vi "Main_Robot_Control.vi"() -> ()   [LabVIEW 2014]
uses:
  <instrlib>/Hokuyo URG Series/Public/Initialize-Standard.vi
  <instrlib>/Hokuyo URG Series/Hokuyo URG Series.lvlib
panel:
  in  "stop 2":bool
  in  "polar attributes (hidden)":T1={"maximum"=30000.0, "minimum"=0.0, "clip to min"=FALSE, "log?(F)"=TRUE, "grid color"=6710886, "plot color"=65280, "fmt and prec"={"format"=enum."Decimal", "precision"=0}, "visible section"=8} {"minimum" format="%0.2f"; "maximum" format="%0.2f"}
  in  "Tab Control":T2(tab)
  out "?":dbl(knob) scale=-800.0..800.0
  out "Sensor Head Position":dbl
  out "Blinky Light":bool
  out "Stop Engaged":bool
  in  "?":bool
  out "Raw Volts":dbl
  out "Center_JR":dbl(slide) scale=0.0..3.0
  out "Pot":dbl(slide) min=0.0 max=5.0 step=0.25 scale=0.0..5.0
  in  "Motor Direction":bool
  in  "1) SET Start Position of Head":dbl
  in  "stop":bool
  out "IR_V":dynamicdata(graph)
  out "Pot_V":dynamicdata(graph)
  out "IR_D":dynamicdata(graph)
  out "Pot_D":dynamicdata(graph)
  out "Data Aquired":picture
  out "Blinky LIDAR  Running":bool
  in  "VISA resource name":refnum<visa-resource-name>="COM3"
  in  "Encoding Width":u16(ring)=3 items=["2 Byte"=2, "3 Byte"=3]
  in  "Cluster Count":dbl=1.0
  in  "Start Point":dbl=-50.0
  in  "End Point":dbl=33.0
  in  "Max (m)":dbl=1.0
  in  "Plot Color":u32(colorbox)=14422272
  in  "Grid Color":u32(colorbox)=11776947
  in  "Stop":bool
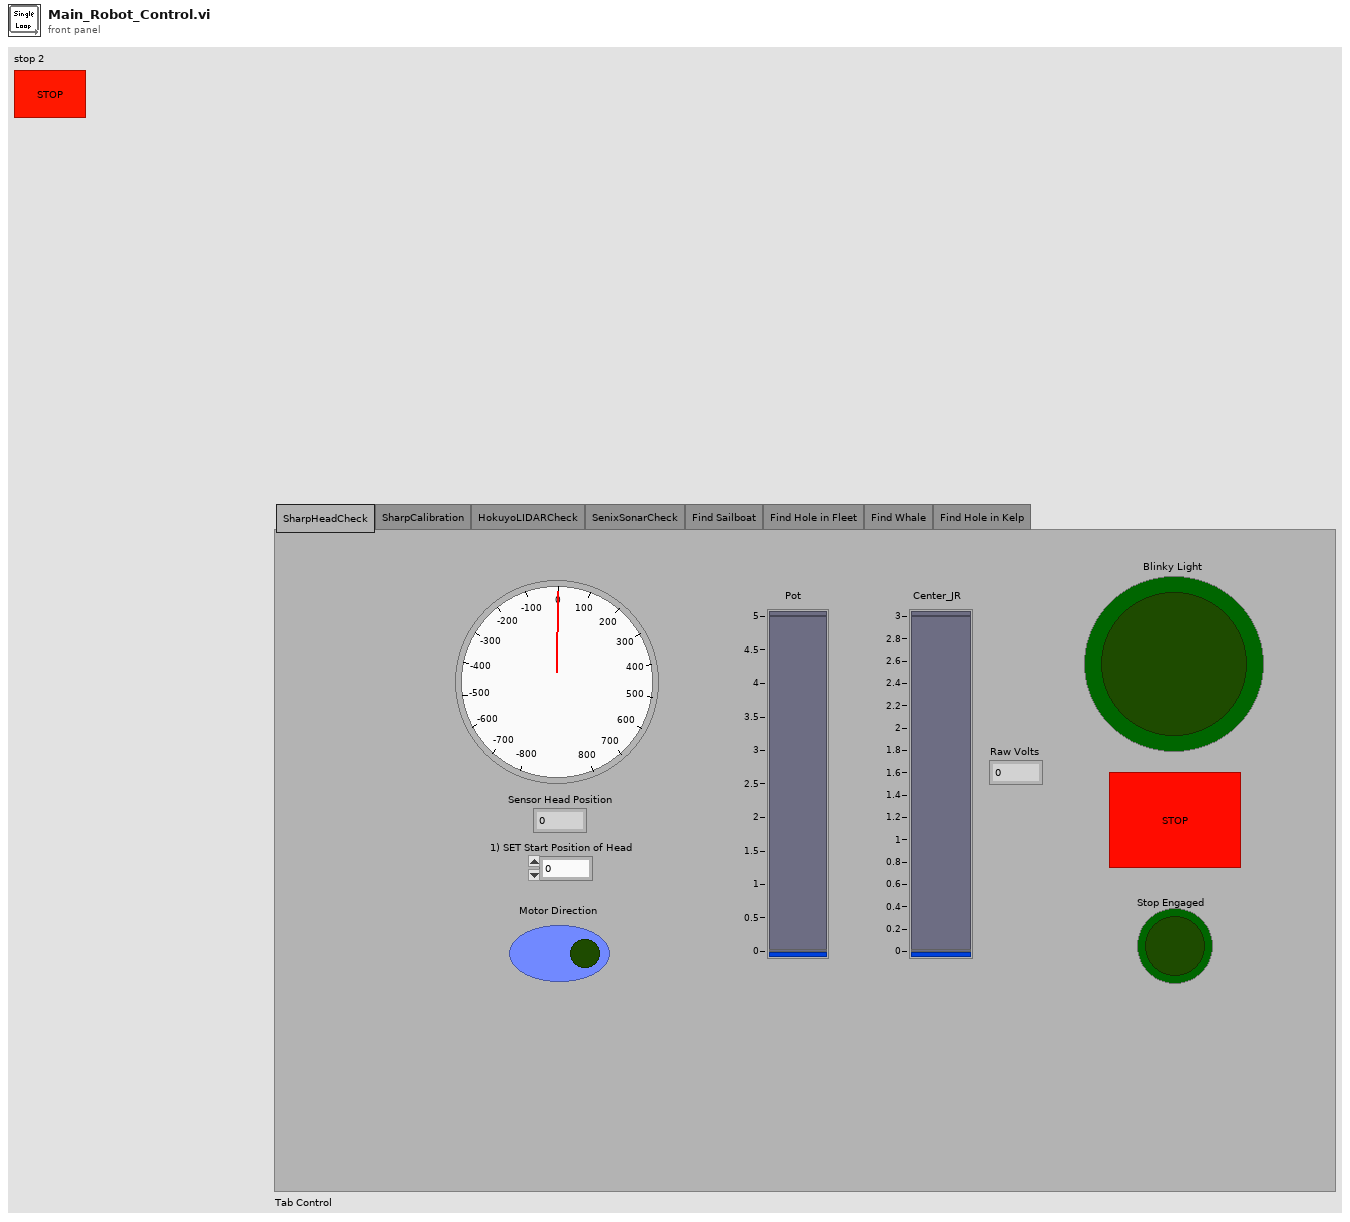
[diagram p1: front panel]
types:
  T1 = cluster{"maximum":dbl, "minimum":dbl, "clip to min":bool, "log?(F)":bool, "grid color":u32, "plot color":u32, "fmt and prec":cluster{"format":enum8{"Decimal", "Scientific", "Engineering", "Binary", "Octal", "Hex"}, "precision":u8}, "visible section":u16}
  T2 = enum32{"SharpHeadCheck", "SharpCalibration", "HokuyoLIDARCheck", "SenixSonarCheck", "Find Sailboat", "Find Hole in Fleet", "Find Whale", "Find Hole in Kelp"}
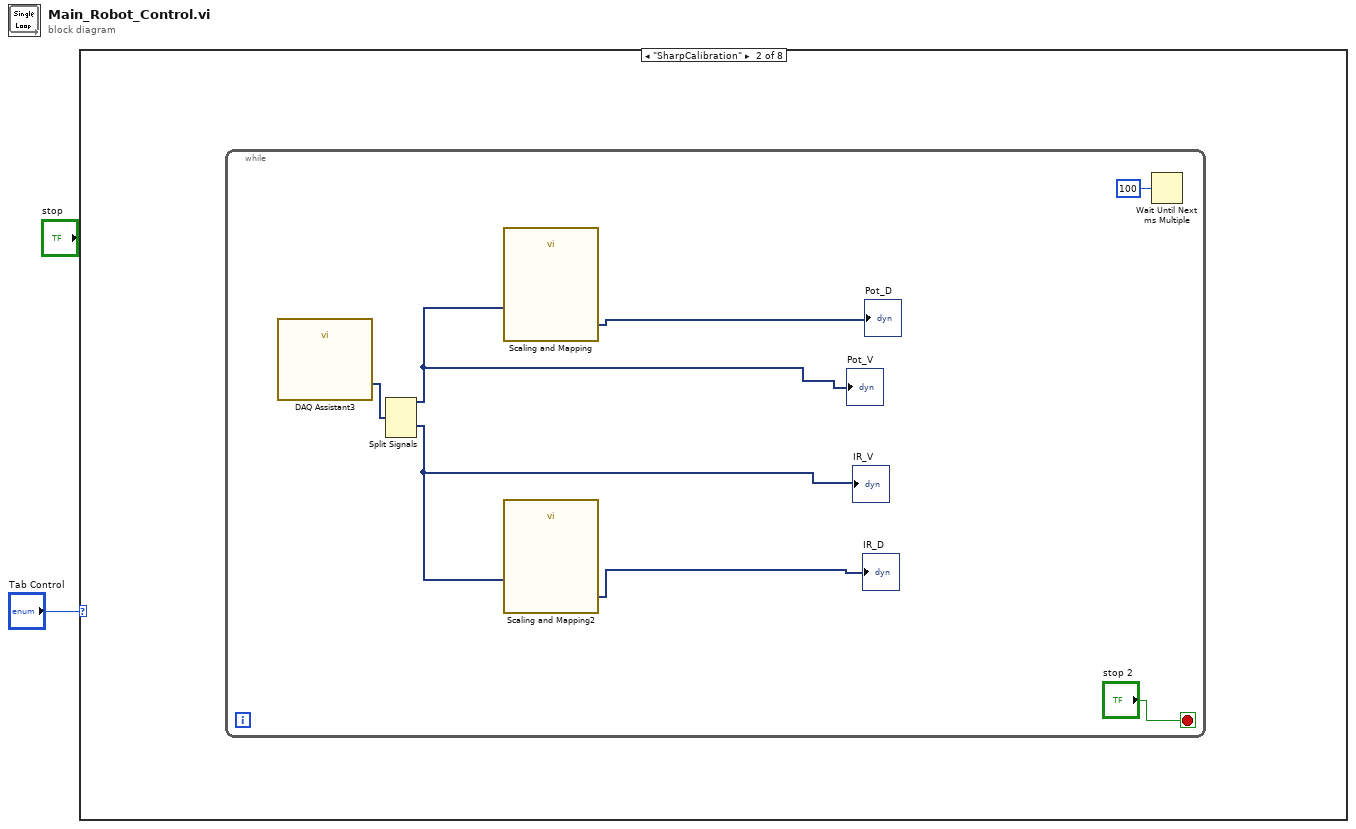
[diagram p0: block diagram]
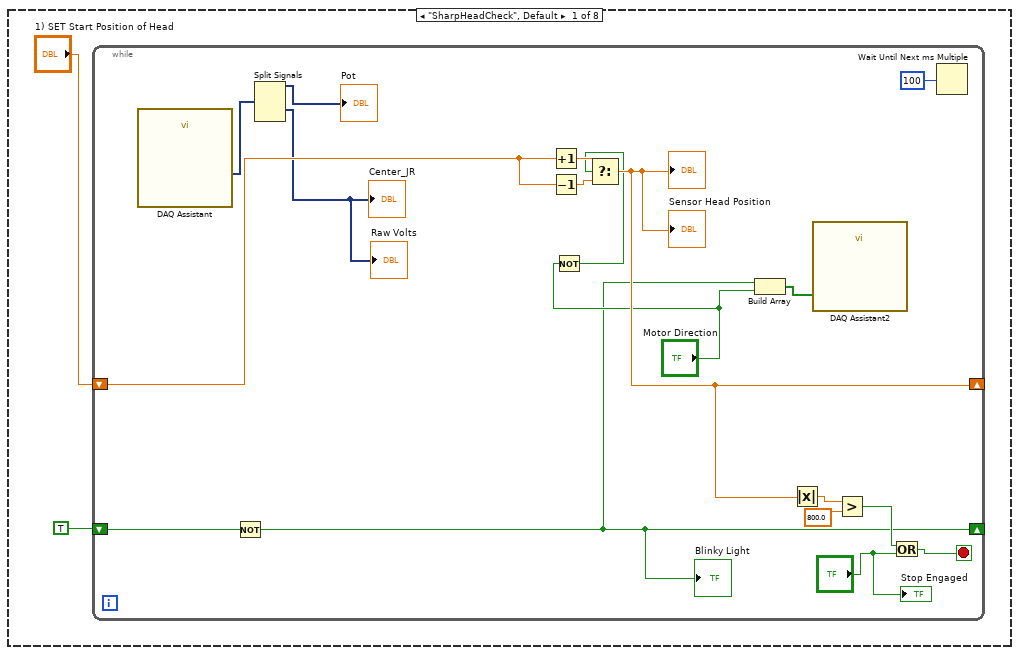
[diagram p2: hidden frame]
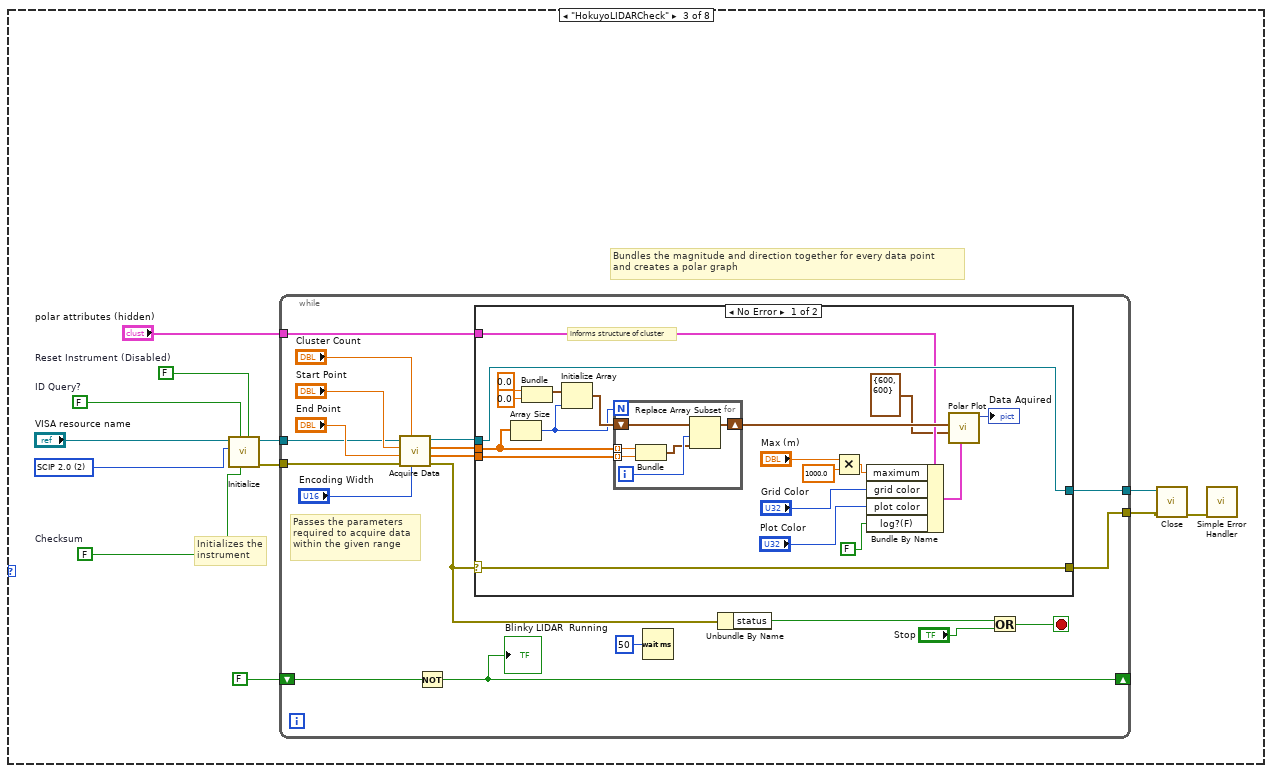
[diagram p3: hidden frame]
diagram:
  n1 = case shown="\"SharpCalibration\"" "Tab Control" {
    frame "SharpHeadCheck", Default {
      n2 = while {
        shift-right: [w12] -> _
        shift-left: "1) SET Start Position of Head" -> [w14]
        shift-right: [w4] -> _
        shift-left: TRUE -> [w5]
        stop <- w21 stop-if-true
        n3 = call "DAQ Assistant"() -> ("data"=w9:dynamicdata)  [unwired: 17 in, 2 out]
        n4 = Not(x=w5) -> (.not. x?=w4:bool)
        "Blinky Light" <- w4
        n5 = Split Signals(w9) -> (→"Pot":dynamicdata, →"Center_JR" →"Raw Volts":dynamicdata)  [unwired: 5 in, 3 out]
        n6 = Increment(x=w14) -> (x+1=w16:dbl)
        n7 = Decrement(x=w14) -> (x-1=w15:dbl)
        n8 = Not(x="Motor Direction") -> (.not. x?=w11:bool)
        n9 = Select(t=w16, s=w11, f=w15) -> (s? t:f=w12:dbl)
        "Sensor Head Position" <- w12
        "?" <- w12
        n10 = Build Array(w4, "Motor Direction") -> (w6:bool[])
        n11 = Absolute Value(x=w12) -> (abs(x)=w17:dbl)
        n12 = call "DAQ Assistant2"("data"=w6) -> ()  [unwired: 17 in, 2 out]
        n13 = Greater?(x=w17, y=800.0) -> (0:w19:bool)
        n14 = Or(x=w19, y="?") -> (x .or. y?=w21:bool)
        n15 = Wait Until Next ms Multiple(millisecond multiple=100) -> ()  [unwired: 1 out]
        "Stop Engaged" <- "?"
      }
    }
    frame "SharpCalibration" {
      n16 = while {
        stop <- "stop 2" stop-if-true
        n17 = call "DAQ Assistant3"() -> ("data"=w26:dynamicdata)  [unwired: 17 in, 2 out]
        n18 = Split Signals(w26) -> (w25:dynamicdata, w24:dynamicdata)  [unwired: 5 in, 3 out]
        "Pot_V" <- w25
        "IR_V" <- w24
        n19 = call "Scaling and Mapping"("Signals"=w25) -> ("Scaled Signals"=→"Pot_D":dynamicdata)  [unwired: 9 in, 1 out]
        n20 = call "Scaling and Mapping2"("Signals"=w24) -> ("Scaled Signals"=→"IR_D":dynamicdata)  [unwired: 9 in, 1 out]
        n21 = Wait Until Next ms Multiple(millisecond multiple=100) -> ()  [unwired: 1 out]
      }
    }
    frame "HokuyoLIDARCheck" {
      w38 = FALSE  # Checksum
      w36 = FALSE  # ID Query?
      w34 = u32 2 items=["Convert to Latest", "SCIP 1.1", "SCIP 2.0"] ("Protocol")
      w35 = FALSE  # Reset Instrument (Disabled)
      # "Bundles the magnitude and direction together for every data point\nand creates a polar graph"
      # "Initializes the instrument"
      n22 = call-poly <instrlib>:"Initialize.vi"("Reset? (F: No)"=w35, "Checksum (Disabled)"=w38, "ID Query? (Enabled)"=w36, "Protocol (2: SCIP 2.0)"=w34, "VISA resource name"="VISA resource name") -> ("error out"=w31:errorcluster, "VISA resource name out"=w32:refnum<visa-resource-name>)  [unwired: 5 in]
      n23 = while {
        tunnel: w32 -> [w47]
        tunnel: [w59] -> w40
        tunnel: [w58] -> w33
        tunnel: w31 -> [w46]
        tunnel: "polar attributes (hidden)" -> [w45]
        shift-right: [w41] -> _
        shift-left: FALSE -> [w42]
        stop <- w55 stop-if-true
        # "Passes the parameters\nrequired to acquire data\nwithin the given range"
        n24 = call <instrlib>:"Acquire Data.vi"("Data Encoding Width (3 Byte)"="Encoding Width", "Cluster Count (1)"="Cluster Count", "error in (no error)"=w46, "End Point (120°)"="End Point", "Start Point (-120°)"="Start Point", "VISA resource name"=w47) -> ("error out"=w51:errorcluster, "Direction"=w52:dbl[], "Magnitude"=w53:dbl[], "VISA resource name out"=w54:refnum<visa-resource-name>)  [unwired: 2 in]
        n25 = Not(x=w42) -> (.not. x?=w41:bool)
        "Blinky LIDAR  Running" <- w41
        n26 = case shown="No Error" w51 {
          selector: w51 -> [w77 w87]
          tunnel: [w77 w87] -> w59
          tunnel: w54 -> [w78 w86]
          tunnel: [w78 w86] -> w58
          tunnel: w53 -> [w72 _]
          tunnel: w52 -> [w71 _]
          tunnel: w45 -> [w67 _]
          frame No Error {
            # "informs structure of cluster"
            n27 = Array Size(array=w72) -> (size(s)=w70:i32)
            n28 = Bundle(0.0, 0.0) -> (w74:cluster{dbl, dbl})  [unwired: 1 in]
            n29 = Initialize Array(w74, w70) -> (w73:cluster{dbl, dbl}[])
            n30 = for {
              N: w70 -> [_]
              shift-right: [w81] -> w69
              shift-left: w73 -> [w82]
              tunnel: w72 -> [w85] mode=indexing
              tunnel: w71 -> [w84] mode=indexing
              i -> [w83]
              n31 = Bundle(w85, w84) -> (w80:cluster{dbl, dbl})  [unwired: 1 in]
              n32 = Replace Array Subset(array=w82, new element=w80, index=w83) -> (w81:cluster{dbl, dbl}[])
            }
            n33 = Multiply(x="Max (m)", y=1000.0) -> (x*y=w63:dbl)
            n34 = Bundle By Name(cluster=w67, "maximum"=w63, "grid color"="Grid Color", "plot color"="Plot Color", "log?(F)"=FALSE) -> (w68:T1)
            n35 = call <vilib>:"Polar Plot.vi"("polar attributes"=w68, "dimensions (w,h)"=cluster{"width":i16, "height":i16} {"width"=600, "height"=600}, "data array [mag, phase (deg)]"=w69) -> ("new picture"=→"Data Aquired":picture)  [unwired: 8 in]
          }
          frame Error {
          }
        }
        n36 = Wait (ms)(milliseconds to wait=u32 50) -> ()  [unwired: 1 out]
        n37 = Unbundle By Name(w51) -> ("status"=w57:bool)
        n38 = Or(x=w57, y="Stop") -> (x .or. y?=w55:bool)
      }
      n39 = call <instrlib>:"Close.vi"("error in (no error)"=w40, "VISA resource name"=w33) -> ("error out"=w37:errorcluster)  [unwired: 9 in]
      n40 = call <vilib>:"Simple Error Handler.vi"("error in (no error)"=w37) -> ()  [unwired: 4 in, 5 out]
    }
    frame "SenixSonarCheck" {
    }
    frame "Find Sailboat" {
    }
    frame "Find Hole in Fleet" {
    }
    frame "Find Whale" {
    }
    frame "Find Hole in Kelp" {
    }
  }
